vi "acquire cursor window data.vi"(6 "start index (0)":i32, 7 "arr action":T1, 9 "z in":cdb[](array[numeric]), 10 "omega in":dbl[](array[numeric]), 11 "cursor window":T2={"left"=2378.60310421286, "right "=2421.6740576496672, "center"=2421.6740576496672, "window"=2421.6740576496672, "cursors"=[], "relative"=0, "absolute"=0, "fixed vertical offset"=2421.6740576496672, "vertical offset"=2421.6740576496672, "skew"=2421.6740576496672, "default window frac"=2421.6740576496672, "kind"=enum."skewed", "skew.left"=2421.6740576496672, "skew.right"=2421.6740576496672, "Plot ref"=refnum, "wing order"=enum."back"}) -> (0 "right index":dbl, 1 "z out":cdb[](array[numeric]), 2 "omega  out":dbl[](array[numeric]), 3 "left index":dbl, 4 "length index":dbl)   [LabVIEW 2020]
uses:
  cursor winow.ctl
  arr action.ctl
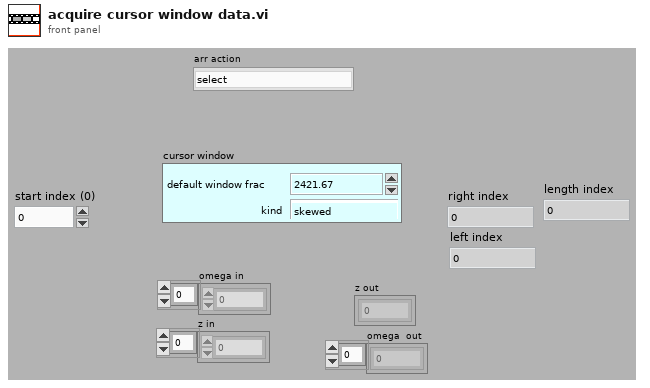
[diagram p1: front panel]
types:
  T1 = typedef "arr action.ctl" = enum16{"select", "remove", "init", "check"}
  T2 = typedef "cursor winow.ctl" = cluster{"left":dbl, "right ":dbl, "center":dbl, "window":dbl, "cursors":i32[], "relative":i32, "absolute":i32, "fixed vertical offset":dbl, "vertical offset":dbl, "skew":dbl, "default window frac":dbl, "kind":enum16{"symmetric", "skewed", "fancy"}, "skew.left":dbl, "skew.right":dbl, "Plot ref":refnum<vi>, "wing order":enum16{"forw", "back"}}
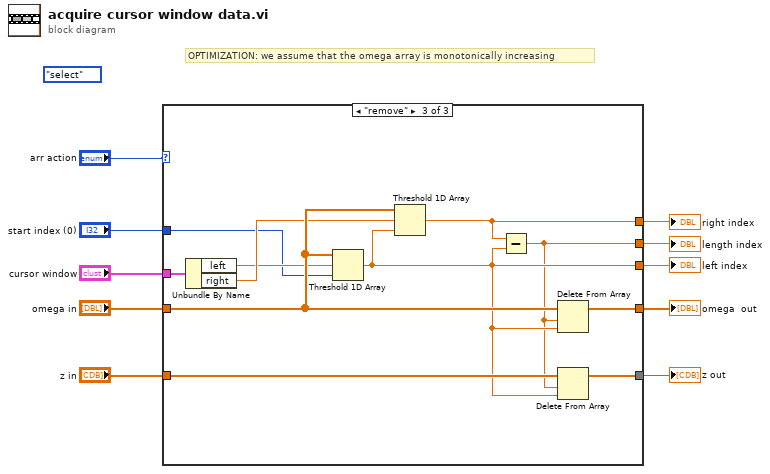
[diagram p0: block diagram]
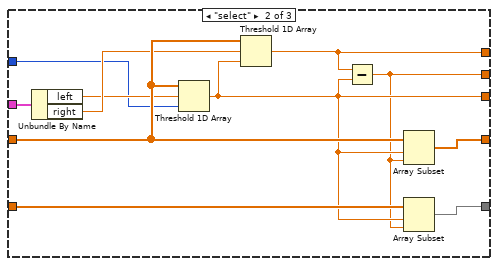
[diagram p3: hidden frame]
diagram:
  (unwired) arr_action."select" ("arr action")
  # "OPTIMIZATION: we assume that the omega array is monotonically increasing"
  n1 = case shown="\"remove\"" "arr action" {
    tunnel: [_ w23 w34] -> w10
    tunnel: "omega in" -> [w11 w22 w33]
    tunnel: [w11 w21 w25] -> w8
    tunnel: "cursor window" -> [_ w20 w32]
    tunnel: "z in" -> [w12 w17 w29]
    tunnel: [w12 w16 w24] -> w5
    tunnel: "start index (0)" -> [_ w15 w28]
    tunnel: [_ w14 w27] -> w3
    tunnel: [_ w13 w26] -> w2
    frame "check", Default {
    }
    frame "select" {
      n2 = Unbundle By Name(w20) -> ("left"=w18:dbl, "right"=w19:dbl)
      n3 = Threshold 1D Array(1:w15, 2:w18, 3:w22) -> (0:w14:dbl)
      n4 = Threshold 1D Array(1:w14, 2:w19, 3:w22) -> (0:w23:dbl)
      n5 = Subtract(x=w23, y=w14) -> (x-y=w13:dbl)
      n6 = Array Subset(array=w22, index=w14, length=w13) -> (w21:dbl[])
      n7 = Array Subset(array=w17, index=w14, length=w13) -> (w16:cdb[])
    }
    frame "remove" {
      n8 = Unbundle By Name(w32) -> ("left"=w30:dbl, "right"=w31:dbl)
      n9 = Threshold 1D Array(1:w28, 2:w30, 3:w33) -> (0:w27:dbl)
      n10 = Threshold 1D Array(1:w27, 2:w31, 3:w33) -> (0:w34:dbl)
      n11 = Subtract(x=w34, y=w27) -> (x-y=w26:dbl)
      n12 = Delete From Array(array=w33, length=w26, index=w27) -> (array with subset deleted=w25:dbl[])  [unwired: 1 out]
      n13 = Delete From Array(array=w29, length=w26, index=w27) -> (array with subset deleted=w24:cdb[])  [unwired: 1 out]
    }
  }
  "z out" <- w5
  "omega  out" <- w8
  "right index" <- w10
  "left index" <- w3
  "length index" <- w2
